vi "Set Overlay Type.vi"(8 "error in (no error)":errorcluster, 10 "Overlay Type":T1, 11 "Element In":refnum<class "Config Element.lvclass">) -> (0 "error out":errorcluster, 3 "Element":refnum<class "Config Element.lvclass">)   [LabVIEW 2020, in "VolatusConfig.lvlib"]
uses:
  lv-cdm/CDM-Config/Config Element/Config Element.lvclass
  Meta Name.ctl
  VolatusConfig.lvlib
  Overlays.ctl
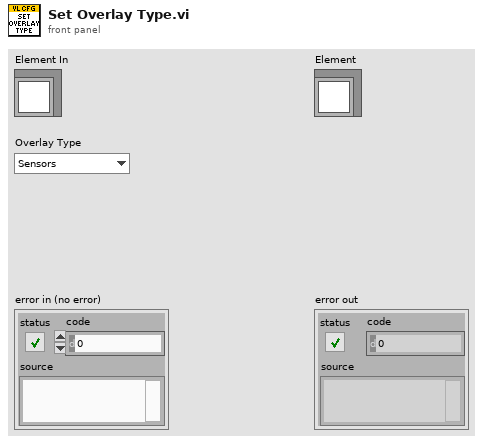
[diagram p1: front panel]
types:
  T1 = typedef "VolatusConfig.lvlib/Overlays.ctl" = enum16{"Sensors", "Wiring"}
  T2 = typedef "VolatusConfig.lvlib/Meta Name.ctl" = enum16{"VL_Type", "VL_Node_IP", "VL_Node_Type", "VL_Task_Type", "VL_Group_Type", "VL_Channel_Type", "VL_Channel_DataType", "VL_Config_Version", "VL_Overlay_Type"}
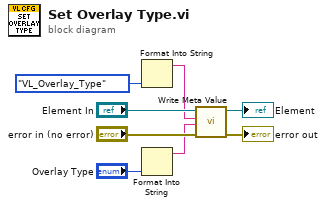
[diagram p0: block diagram]
diagram:
  n1 = Format Into String(Meta_Name."VL_Overlay_Type" ("Meta Name")) -> (resulting string=w3:string)  [unwired: 3 in, 1 out]
  n2 = Format Into String("Overlay Type") -> (resulting string=w2:string)  [unwired: 3 in, 1 out]
  n3 = call "Write Meta Value.vi"("error in (no error)"="error in (no error)", "Meta Value"=w2, "Meta Name"=w3, "Config Element in"="Element In") -> ("error out"=→"error out":errorcluster, "Config Element out"=→"Element":refnum<class "Config Element.lvclass">)  [unwired: 6 in]
